vi "TBQ_QueueFull.vi"(11 "TBQ In":refnum<class "TimeBasedQueue.lvclass">) -> (1 "Queue Full?":bool, 3 "TBQ Out":refnum<class "TimeBasedQueue.lvclass">)   [LabVIEW 2012, in "TimeBasedQueue.lvclass"]
uses:
  TimeBasedQueue.lvclass
  TimeBasedQueue.lvclass/TimeBasedQueue.ctl
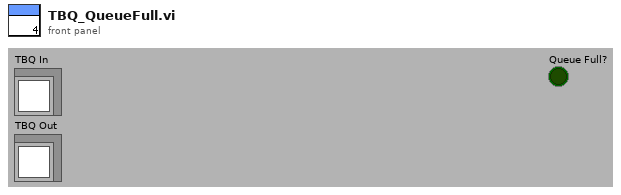
[diagram p1: front panel]
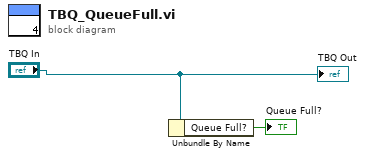
[diagram p0: block diagram]
diagram:
  n1 = Unbundle By Name("TBQ In") -> ("Queue Full?"=→"Queue Full?":bool)
  "TBQ Out" <- "TBQ In"
